vi "Disconnect.vi"(8 "error in (no error)":errorcluster, 11 "TC01 in":refnum<class "TC01T.lvclass">) -> (0 "error out":errorcluster, 3 "TC01 out":refnum<class "TC01T.lvclass">)   [LabVIEW 2018, in "TC01T.lvlib" / "TC01T.lvclass"]
uses:
  TC01T.lvclass
  builds/Thermocouple.lvlibp/Thermocouple.lvclass
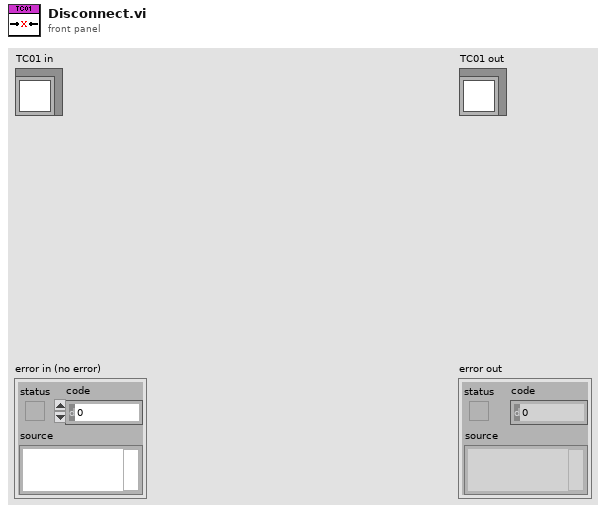
[diagram p1: front panel]
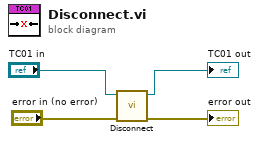
[diagram p0: block diagram]
diagram:
  n1 = call-parent "Disconnect.vi"("error in (no error)"="error in (no error)", "Thermocouple in"="TC01 in") -> ("error out"=→"error out":errorcluster, "Thermocouple out"=→"TC01 out":refnum<class "TC01T.lvclass">)  [unwired: 8 in]
